vi "Clear Set.vi"(0 "DBSet in":refnum<class "DBSet.lvclass">, 11 "error in (no error)":errorcluster {"code" format="Error %.0f"}) -> (4 "DBSet out":refnum<class "DBSet.lvclass">, 15 "error out":errorcluster {"code" format="Error %.0f"})   [LabVIEW 2024, in "DBSet.lvclass"]
uses:
  DBSet.lvclass
  DBSet.lvclass/DBSet.ctl
  <vilib>/drjdpowell/SQLite Library/SQLite.lvlib
  <vilib>/drjdpowell/SQLite Library/SQL Connection/Execute SQL (Single Integer).vi
  <vilib>/drjdpowell/SQLite Library/SQL Connection/Connection.lvclass
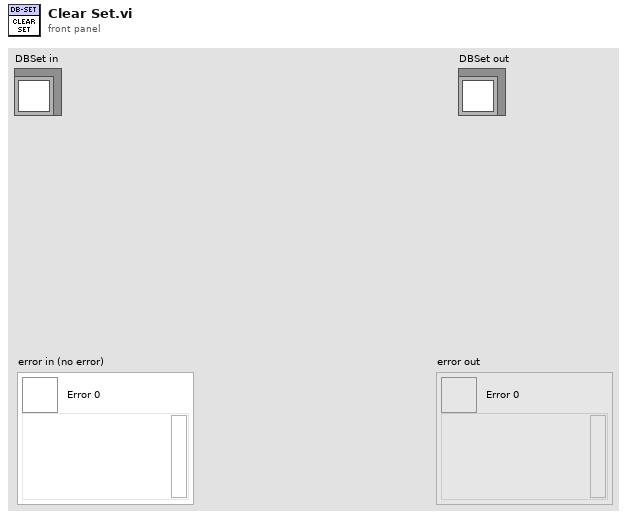
[diagram p1: front panel]
types:
  T1 = typedef "Semaphore RefNum" = refnum<k1>
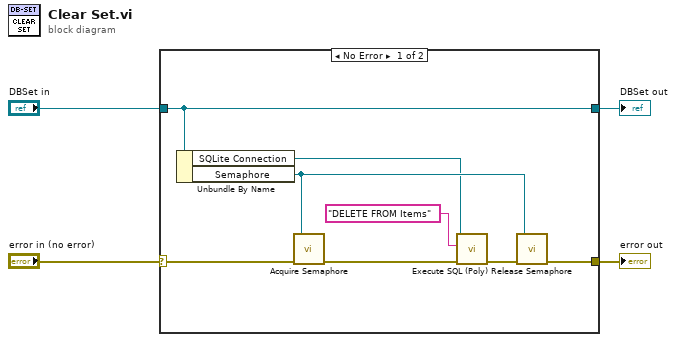
[diagram p0: block diagram]
diagram:
  n1 = case shown="No Error" "error in (no error)" {
    selector: "error in (no error)" -> [w11 w14]
    tunnel: [w10 w14] -> w3
    tunnel: [w12 w13] -> w1
    tunnel: "DBSet in" -> [w12 w13]
    frame No Error {
      n2 = Unbundle By Name(w12) -> ("SQLite Connection"=w5:refnum<class "Connection.lvclass">, "Semaphore"=w9:T1)
      n3 = call <vilib>:"Acquire Semaphore.vi"("error in (no error)"=w11, "semaphore"=w9) -> ("error out"=w7:errorcluster)  [unwired: 3 in, 2 out]
      n4 = call-poly <vilib>:"Execute SQL (Poly).vi"("error in (no error)"=w7, "SQL"="DELETE FROM Items", "SQLite Connection in"=w5) -> ("error out"=w6:errorcluster)  [unwired: 6 in, 2 out]
      n5 = call <vilib>:"Release Semaphore.vi"("error in (no error)"=w6, "semaphore"=w9) -> ("error out"=w10:errorcluster)  [unwired: 4 in, 1 out]
    }
    frame Error {
    }
  }
  "error out" <- w3
  "DBSet out" <- w1
